vi "Sine Wave Generator [Software-Timed].vi"() -> ()   [LabVIEW 2017]
uses:
  <vilib>/imath/engines/lvmath2/RunTimeEngine/Managers/WorkSpace/UID Generator.vi
  <vilib>/imath/engines/lvmath2/RunTimeEngine/RunTimeType/NIMS_RunTimeType_From StrictType (excl LVString).vi
  <instcachedir>/0/NIMS_RunTimeType_From StrictType (excl LVString)_1019F277F0A747EDBCA0F6C52CA54500.lvgen/NIMS_RunTimeType_From StrictType (excl LVString)_1019F277F0A747EDBCA0F6C52CA54500_000.vi
  <vilib>/imath/engines/lvmath2/RunTimeEngine/LocalVariableDefStatement/MC_LocalVariableDefStatement_Display.vi
  <vilib>/imath/engines/lvmath2/RunTimeEngine/Managers/SymbolTable/Clear UID.vi
  <vilib>/imath/engines/lvmath2/RunTimeEngine/NodeEndStatement/NIMS_NodeEndStatement_Output.vi
  <instcachedir>/0/NIMS_NodeEndStatement_Output_53EC0D466D134D7ABD903AC30B43404B.lvgen/NIMS_NodeEndStatement_Output_53EC0D466D134D7ABD903AC30B43404B_001.vi
  <vilib>/imath/engines/lvmath2/RunTimeEngine/ErrorHandling/NIMS_Finalize Error.vi
  <vilib>/imath/engines/lvmath2/RunTimeEngine/Managers/SymbolTable/NIMS_WorkSpace.lvlib
panel:
  out "Waveform Chart":dbl(graph)
  out "error out":errorcluster
  in  "Samples per Cycle":dbl=100.0 format="%.4g"
  in  "stop":bool
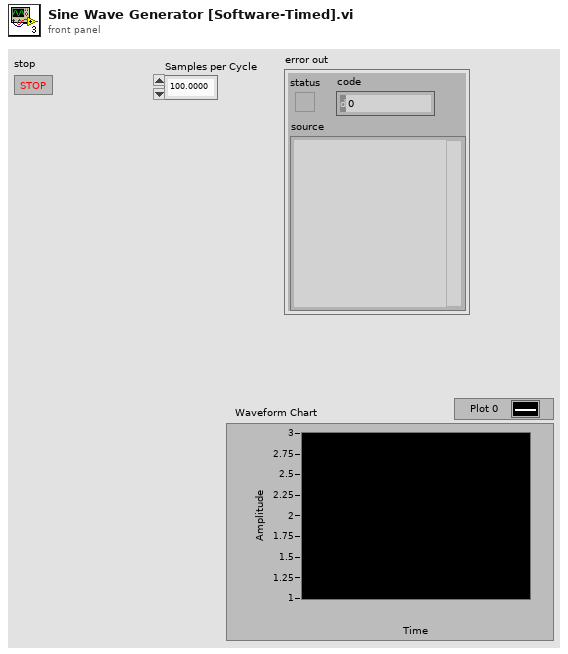
[diagram p1: front panel]
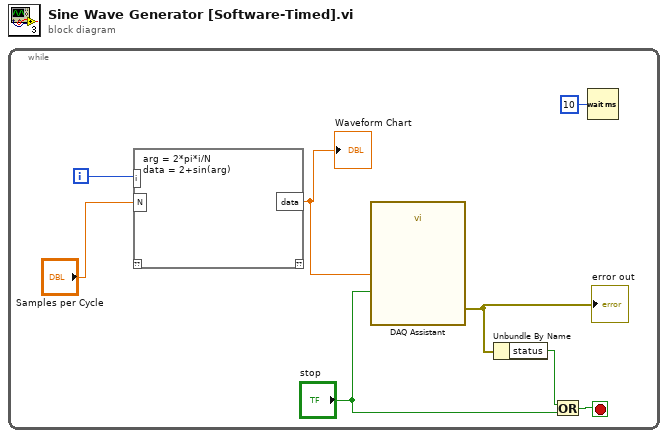
[diagram p0: block diagram]
diagram:
  n1 = while {
    i -> [w3]
    stop <- w4 stop-if-true
    n2 = mathscript code="arg = 2*pi*i/N\ndata = 2+sin(arg)"("i"=w3, "N"="Samples per Cycle") -> ("data"=w1:dbl)  [unwired: 1 in, 1 out]
    "Waveform Chart" <- w1
    n3 = call "DAQ Assistant"("data"=w1, "stop (T)"="stop") -> ("error out"=w7:errorcluster)  [unwired: 16 in, 1 out]
    "error out" <- w7
    n4 = Unbundle By Name "Unbundle By Name"(w7) -> ("status"=w5:bool)
    n5 = Or(x=w5, y="stop") -> (x .or. y?=w4:bool)
    n6 = Wait (ms)(milliseconds to wait=u32 10) -> ()  [unwired: 1 out]
  }
